vi "Create Log Data.vi"(8 "error in (no error)":errorcluster, 9 "System Time":dbl[](array[numeric]), 10 "Actual Values":dbl[][](array[numeric]), 11 "Test Data":T1[](array[typedef])) -> (0 "error out":errorcluster, 1 "Log Data":string[][](array[string]))   [LabVIEW 2011]
uses:
  Controls/Test Column Data.ctl
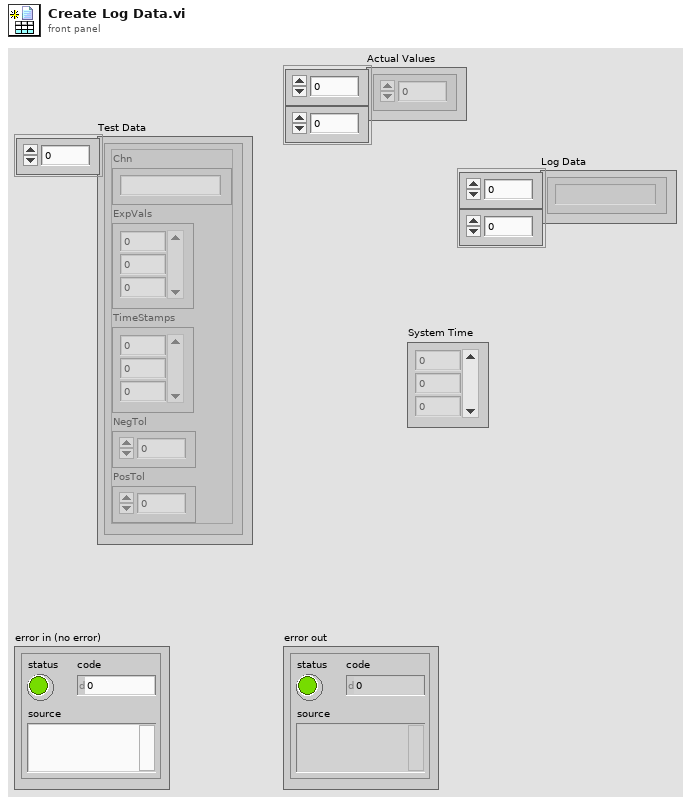
[diagram p1: front panel]
types:
  T1 = typedef "Test Column Data.ctl" = cluster{"Chn":string, "ExpVals":dbl[], "TimeStamps":i64[], "NegTol":dbl, "PosTol":dbl}
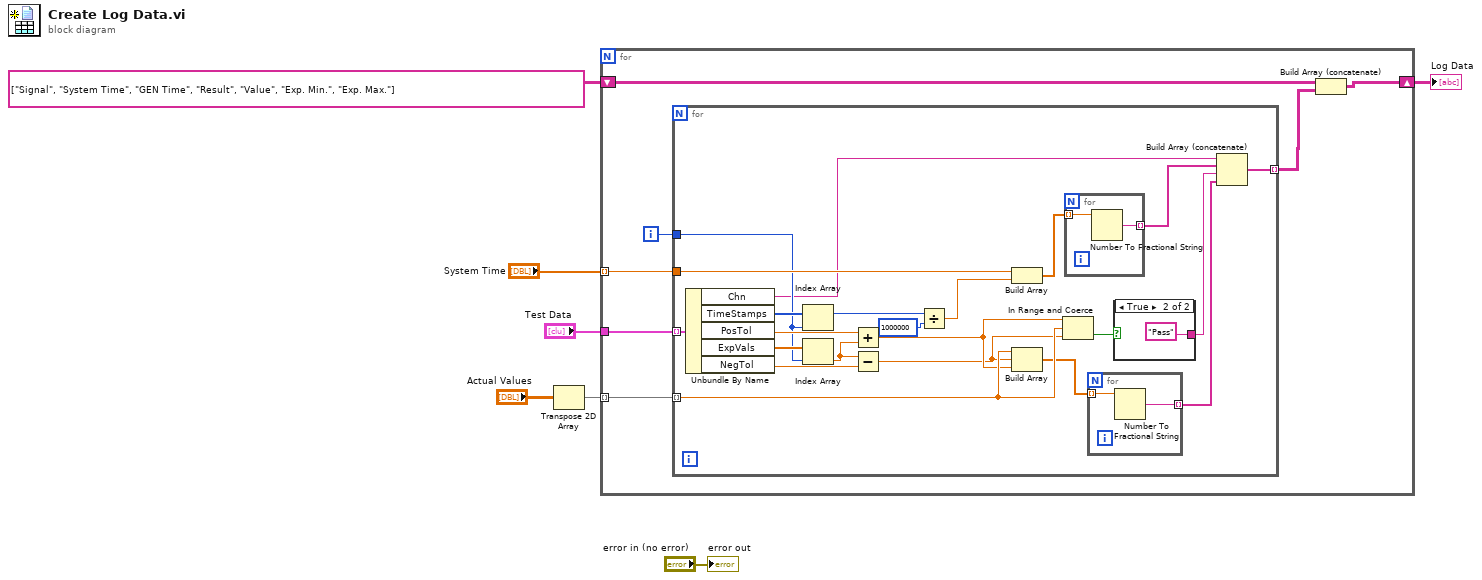
[diagram p0: block diagram]
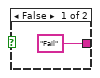
[diagram p2: hidden frame]
diagram:
  n1 = Transpose 2D Array(2D array="Actual Values") -> (transposed array=w1:dbl[][])
  n2 = for {
    tunnel: "Test Data" -> [w10]
    tunnel: w1 -> [w14] mode=indexing
    tunnel: "System Time" -> [w13] mode=indexing
    shift-right: [w11] -> w3
    shift-left: string[][] [["Signal", "System Time", "GEN Time", "Result", "Value", "Exp. Min.", "Exp. Max."]] -> [w12]
    i -> [w9]
    n3 = for {
      tunnel: w14 -> [w35] mode=indexing
      tunnel: w13 -> [w36]
      tunnel: w10 -> [w24] mode=indexing
      tunnel: w9 -> [w21]
      tunnel: [w15] -> w8 mode=indexing
      n4 = Unbundle By Name(w24) -> ("Chn"=w19:string, "TimeStamps"=w26:i64[], "PosTol"=w28:dbl, "ExpVals"=w22:dbl[], "NegTol"=w27:dbl)
      n5 = Index Array(array=w26, index=w21) -> (element=w23:i64)
      n6 = Index Array(array=w22, index=w21) -> (element=w20:dbl)
      n7 = Add(x=w28, y=w20) -> (x+y=w17:dbl)
      n8 = Subtract(x=w20, y=w27) -> (x-y=w16:dbl)
      n9 = Divide(x=w23, y=i64 1000000 ("x")) -> (x/y=w18:dbl)
      n10 = Build Array(w36, w18) -> (w33:dbl[])
      n11 = Build Array(w35, w16, w17) -> (w34:dbl[])
      n12 = In Range and Coerce(upper limit=w17, x=w35, lower limit=w16) -> (In Range?=w31:bool)  [unwired: 1 out]
      n13 = for {
        tunnel: w33 -> [w40] mode=indexing
        tunnel: [w39] -> w32 mode=indexing
        n14 = Number To Fractional String(number=w40) -> (F-format string=w39:string)  [unwired: 3 in]
      }
      n15 = for {
        tunnel: w34 -> [w42] mode=indexing
        tunnel: [w41] -> w29 mode=indexing
        n16 = Number To Fractional String(number=w42) -> (F-format string=w41:string)  [unwired: 3 in]
      }
      n17 = case shown="True" w31 {
        tunnel: ["Fail" "Pass"] -> w30
        frame False {
        }
        frame True {
        }
      }
      n18 = Build Array (concatenate)(w19, w32, w30, w29) -> (w15:string[])
    }
    n19 = Build Array (concatenate)(w12, w8) -> (w11:string[][])
  }
  "Log Data" <- w3
  "error out" <- "error in (no error)"
